vi "Units_RadiansToRotations.vi"(10 "Radians":dbl) -> (2 "Rotations":dbl)   [LabVIEW 2019, in "Trajectory_Library.lvlib"]
doc: "Convert a angle value from rotations to degrees\n\nInputs: \n - Rotations - Angle (Rotations)\n\nOutputs:\n - Degrees - Angle (Degrees)"
uses:
  Trajectory_Library.lvlib
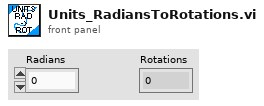
[diagram p1: front panel]
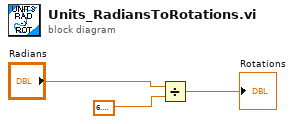
[diagram p0: block diagram]
diagram:
  n1 = Divide(x="Radians", y=6.283185307179586) -> (x/y=→"Rotations":dbl)
